vi "Host Test.vi"() -> ()   [LabVIEW 2012]
uses:
  <vilib>/FPGAPlugInAG/PCI-7831R/niLvFpga_Open_PCI-7831R.vi
  <vilib>/rvi/interface/common/dynamic/niFpgaDynamicAddResources.vi
  <vilib>/Utility/error.llb/Error Cluster From Error Code.vi
  <vilib>/rvi/errors/niLvFpgaAdjustHostInterfaceError.vi
  <vilib>/FPGAPlugInAG/Dynamic/niLvFpga_Close_Dynamic.vi
  <vilib>/rvi/interface/nirviOpenFPGA/nirviOpenFPGA.xnode
  SB130-XPS/Documents/FPGA-project-apporach-retraction/FPGA Bitfiles/Apporach-Retract_FPGATarget2_TargetTest_luhszpaEPZQ.lvbitx
  Target Test.vi
  <vilib>/rvi/interface/nirviReadWriteControl/nirviReadWriteControl.xnode
  <vilib>/rvi/interface/nirviCloseFPGA/nirviCloseFPGA.xnode
  <vilib>/rvi/interface/nirviMethod/nirviMethod.xnode
  NiFpgaLv.dll
  <vilib>/rvi/interface/Simulation/niFpgaSimulationCallBeginRW.vi
  <vilib>/FPGAPlugInAG/Dynamic/niLvFpga_ReadFifo_Dynamic.vi
  <vilib>/rvi/errors/niLvFpgaMergeErrorWithErrorCode.vi
panel:
  out "FPGA Output Voltage":i32[](graph)
  in  "Elements":i32
  in  "Digital Step":i32=640
  out "Control Voltage In Range":bool
  out "Control Voltage Host Indicator":i32
  in  "Control Voltage":i32
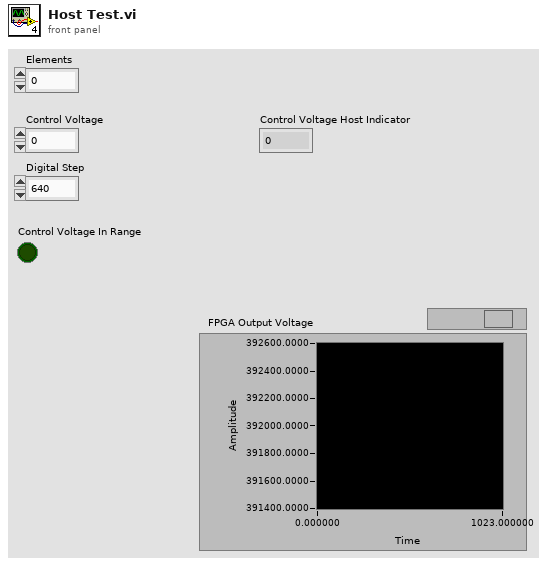
[diagram p1: front panel]
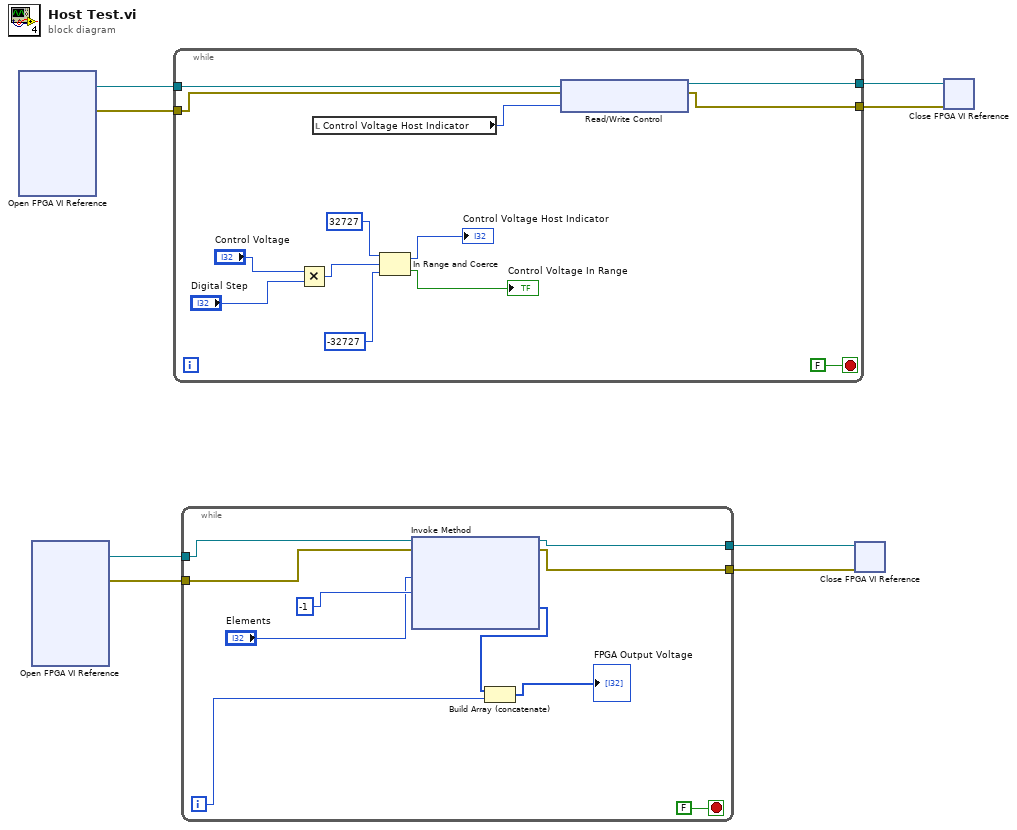
[diagram p0: block diagram]
diagram:
  n1 = xnode "Open FPGA VI Reference"() -> ("FPGA VI Reference Out"=w7:refnum<k20>, "error out"=w8:errorcluster)  [unwired: 2 in]
  n2 = xnode "Open FPGA VI Reference"() -> ("FPGA VI Reference Out"=w4:refnum<k20>, "error out"=w3:errorcluster)  [unwired: 2 in]
  n3 = while {
    tunnel: w7 -> [w13]
    tunnel: w8 -> [w12]
    tunnel: [w11] -> w6
    tunnel: [w10] -> w5
    stop <- FALSE stop-if-true
    n4 = Multiply(x="Control Voltage", y="Digital Step") -> (x*y=w18:i32)
    n5 = local read "Control Voltage Host Indicator"() -> (w9:i32)
    n6 = In Range and Coerce(upper limit=32727, x=w18, lower limit=-32727) -> (coerced(x)=→"Control Voltage Host Indicator":i32, In Range?=→"Control Voltage In Range":bool)
    n7 = xnode "Read/Write Control"("FPGA VI Reference In"=w13, "error in"=w12, "Host Output Voltage"=w9) -> ("FPGA VI Reference Out"=w11:refnum<k20>, "error out"=w10:errorcluster)
  }
  n8 = while {
    tunnel: w4 -> [w30]
    tunnel: w3 -> [w29]
    tunnel: [w28] -> w2
    tunnel: [w27] -> w1
    i -> [w23]
    stop <- FALSE stop-if-true
    n9 = xnode "Invoke Method"("FPGA VI Reference In"=w30, "error in"=w29, "Number of Elements"="Elements", "Timeout (ms)"=-1) -> ("FPGA VI Reference Out"=w28:refnum<k20>, "error out"=w27:errorcluster, "Data"=w22:i16[])  [unwired: 1 out]
    n10 = Build Array (concatenate)(w22, w23) -> (→"FPGA Output Voltage":i32[])
  }
  n11 = xnode "Close FPGA VI Reference"("FPGA VI Reference In"=w2, "error in"=w1) -> ()  [unwired: 1 out]
  n12 = xnode "Close FPGA VI Reference"("FPGA VI Reference In"=w6, "error in"=w5) -> ()  [unwired: 1 out]
